vi "ModifyProjectDeployLVAddons.vi"() -> ()   [LabVIEW 2021]
uses:
  <vilib>/Utility/sysdir.llb/System Directory Type.ctl
  <vilib>/Wiresmith Technology/G CLI/CLI Class/CLI.lvclass
panel:
  out "Custom Parameters":string[](array[string])
  out "error out":errorcluster
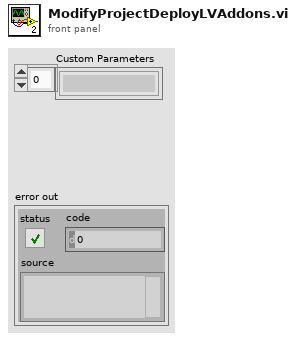
[diagram p1: front panel]
types:
  T1 = typedef "System Directory Type.ctl" = i32
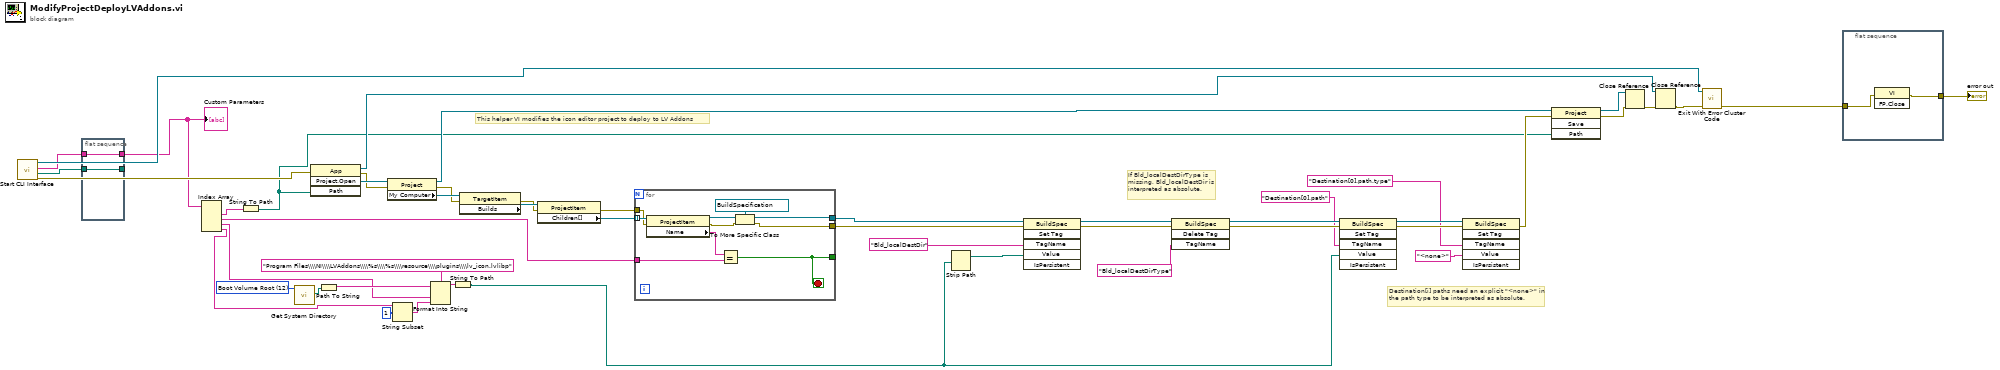
[diagram p0: block diagram]
diagram:
  w10 = T1 12 items=["User Home"=0, "User Desktop"=1, "User Documents"=2, "User Application Data"=3, "User Preferences"=4, "User Temporary"=5, "Public Documents"=6, "Public Application Data"=7, "Public Preferences"=8, "Public Cache"=13, "System Core Libraries"=9, "System Installed Libraries"=10, "Application Files"=11, "Boot Volume Root"=12] ("system directory type")
  # "Destination[i] paths need an explicit \"<none>\" in the path type to be interpreted as absolute."
  # "If Bld_localDestDirType is missing, Bld_localDestDir is interpreted as absolute."
  # "This helper VI modifies the icon editor project to deploy to LV Addons"
  n1 = call <vilib>:"Start CLI Interface.vi"() -> ("error out"=w21:errorcluster, "Working Directory"=w16:path, "Custom Parameters"=w15:string[], "CLI out"=w19:refnum<class "CLI.lvclass">)  [unwired: 8 in]
  n2 = flat-sequence {
    tunnel: w16 -> [w51]
    tunnel: [w51] -> _
    tunnel: w15 -> [w50]
    tunnel: [w50] -> w14
    frame #0 {
    }
  }
  n3 = Index Array(array=w14) -> (element #1=w13:string, element #2=w11:string, element #3=w3:string, element #4=w2:string)  [unwired: 4 in]
  n4 = String To Path(string=w13) -> (path=w12:path)
  n5 = call <vilib>:"Get System Directory.vi"("system directory type"=w10) -> ("system directory"=w5:path)  [unwired: 10 in]
  n6 = invoke class="App" method="Project.Open"(error in=w21, "Path"=w12) -> (reference out=w22:refnum<vi>, error out=w29:errorcluster, "Project:Open"=w44:refnum<vi>)  [unwired: 2 in, 1 out]
  n7 = Path To String(path=w5) -> (string=w4:string)
  n8 = property class="Project"(reference=w44, error in=w29) -> (reference out=w43:refnum<vi>, error out=w28:errorcluster, "My Computer"=w49:refnum<vi>)
  n9 = String Subset(string=w2, offset (0)=1) -> (substring=w7:string)  [unwired: 1 in]
  n10 = Format Into String(format string="Program Files\\\\NI\\\\LVAddons\\\\%s\\\\%s\\\\resource\\\\plugins\\\\lv_icon.lvlibp", initial string=w4, w3, w7) -> (resulting string=w6:string)  [unwired: 1 in, 1 out]
  n11 = String To Path(string=w6) -> (path=w1:path)
  n12 = property class="TargetItem"(reference=w49, error in=w28) -> (error out=w27:errorcluster, "Builds"=w47:refnum<vi>)  [unwired: 1 out]
  n13 = property class="ProjectItem"(reference=w47, error in=w27) -> (error out=w26:errorcluster, "Children[]"=w48:refnum<vi>[])  [unwired: 1 out]
  n14 = for {
    tunnel: w48 -> [w61] mode=indexing
    tunnel: [w54] -> w46
    tunnel: w11 -> [w59]
    tunnel: [w58] -> _
    tunnel: [w55] -> w45
    tunnel: w26 -> [w52]
    stop <- w58 stop-if-true
    n15 = property class="ProjectItem"(reference=w61, error in=w52) -> (reference out=w56:refnum<vi>, error out=w57:errorcluster, "Name"=w60:string)
    n16 = Equal?(x=w60, y=w59) -> (x = y?=w58:bool)
    n17 = To More Specific Class(target class=refnum<vi> refnum ("Build Spec"), reference=w56, error in=w57) -> (specific class reference=w54:refnum<vi>, error out=w55:errorcluster)
  }
  n18 = Strip Path(path=w1) -> (stripped path=w30:path)  [unwired: 1 out]
  n19 = invoke class="BuildSpec" method="Set Tag"(reference=w46, error in=w45, "TagName"="Bld_localDestDir" ("Tag Name"), "Value"=w30) -> (reference out=w42:refnum<vi>, error out=w38:errorcluster)  [unwired: 2 in, 4 out]
  n20 = invoke class="BuildSpec" method="Delete Tag"(reference=w42, error in=w38, "TagName"="Bld_localDestDirType" ("Tag Name")) -> (reference out=w41:refnum<vi>, error out=w37:errorcluster)  [unwired: 1 in, 2 out]
  n21 = invoke class="BuildSpec" method="Set Tag"(reference=w41, error in=w37, "TagName"="Destination[0].path" ("format string"), "Value"=w1) -> (reference out=w36:refnum<vi>, error out=w35:errorcluster)  [unwired: 2 in, 4 out]
  n22 = invoke class="BuildSpec" method="Set Tag"(reference=w36, error in=w35, "TagName"="Destination[0].path.type" ("format string"), "Value"="<none>") -> (error out=w31:errorcluster)  [unwired: 2 in, 5 out]
  n23 = invoke class="Project" method="Save"(reference=w43, error in=w31, "Path"=w12) -> (reference out=w24:refnum<vi>, error out=w25:errorcluster)  [unwired: 1 in, 2 out]
  n24 = Close Reference(reference=w24, error in (no error)=w25) -> (error out=w23:errorcluster)
  n25 = Close Reference(reference=w22, error in (no error)=w23) -> (error out=w20:errorcluster)
  n26 = call <vilib>:"Exit With Error Cluster Code.vi"("error in (no error)"=w20, "CLI in"=w19) -> ("error out"=w18:errorcluster)  [unwired: 9 in]
  n27 = flat-sequence {
    tunnel: [w63] -> w17
    tunnel: w18 -> [w62]
    frame #0 {
      n28 = invoke class="VI" method="FP.Close"(error in=w62) -> (error out=w63:errorcluster)  [unwired: 2 in, 2 out]
    }
  }
  "error out" <- w17
  "Custom Parameters" <- w14
